vi "Adatbevitel.vi"(8 "Error In":errorcluster, 11 "Felhasználói adatok in":T1={"NÉV:"="", "Jelszó: (csak számjegyek)"="", "Felhasználói szint"="Operátor"}) -> (0 "Error Out":errorcluster, 2 "OK ?":bool, 3 "Felhasználói adatok out":string[](array[string]))   [LabVIEW 2014]
panel:
  out "Hibás jelszó":string
  in  "Cancel Button":bool
  in  "OK Button":bool
  # "Új felhasználó adatai"
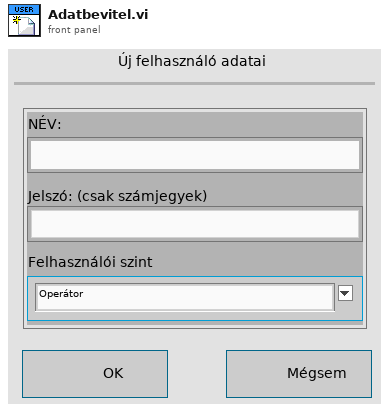
[diagram p1: front panel]
types:
  T1 = typedef "Felhasználó típus.ctl" = cluster{"NÉV:":string, "Jelszó: (csak számjegyek)":string, "Felhasználói szint":string}
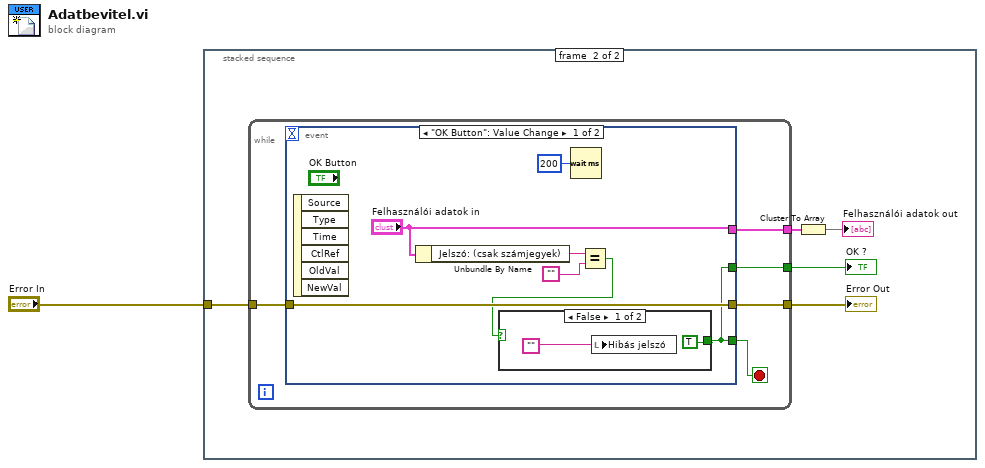
[diagram p0: block diagram]
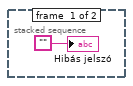
[diagram p2: hidden frame]
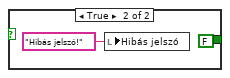
[diagram p3: hidden frame]
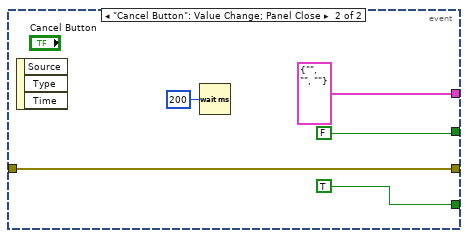
[diagram p4: hidden frame]
diagram:
  n1 = stacked-sequence {
    tunnel: "Error In" -> [_ w7]
    frame #0 {
      "Hibás jelszó" <- ""
    }
    frame #1 {
      n2 = while {
        tunnel: [w12] -> w5
        tunnel: w7 -> [w10]
        tunnel: [w9] -> w6
        tunnel: [w8] -> w3
        stop <- w11 stop-if-true
        n3 = event shown="[0] \"OK Button\": Value Change" {
          selector: _ -> [_ _]
          dyn-events: _ -> [_ _]
          timeout: _ -> [_ _]
          tunnel: ["Felhasználói adatok in" T1 {"NÉV:"="", "Jelszó: (csak számjegyek)"="", "Felhasználói szint"=""} ("Felhasználói adatok in")] -> w12
          tunnel: [w13 TRUE] -> w11
          tunnel: [w18 w25] -> w9
          tunnel: w10 -> [w18 w25]
          tunnel: [w13 FALSE] -> w8
          event "OK Button": Value Change {
            n4 = event-data() -> ()  [unwired: 1 in, 6 out]
            n5 = Unbundle By Name("Felhasználói adatok in") -> ("Jelszó: (csak számjegyek)"=w16:string)
            n6 = Wait (ms)(milliseconds to wait=u32 200) -> ()  [unwired: 1 out]
            n7 = Equal?(x=w16, y="") -> (x = y?=w14:bool)
            n8 = case shown="False" w14 {
              tunnel: [TRUE FALSE] -> w13
              frame False {
                n9 = local write "Hibás jelszó"("") -> ()
              }
              frame True {
                n10 = local write "Hibás jelszó"("Hibás jelszó!" ("Hibás jelszó")) -> ()
              }
            }
          }
          event "Cancel Button": Value Change; Panel Close {
            n11 = event-data() -> ()  [unwired: 1 in, 3 out]
            n12 = Wait (ms)(milliseconds to wait=u32 200) -> ()  [unwired: 1 out]
          }
        }
      }
      "Error Out" <- w6
      "OK ?" <- w3
      n13 = Cluster To Array(cluster=w5) -> (array=→"Felhasználói adatok out":string[])
    }
  }
